vi "Set DataArray.vi"   [LabVIEW 2016, in "DataGrid.lvlib" / "DataGridView.lvclass"]
uses:
  <userlib>/LabVIEWdotNetDataGrid/source/DataGridView/DataGridView.lvclass
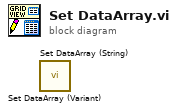
[diagram p0: block diagram]
diagram:
  n1 = call <userlib>:"Set DataArray (String).vi"() -> ()  [unwired: 10 in, 2 out]
  n2 = call <userlib>:"Set DataArray (Variant).vi"() -> ()  [unwired: 10 in, 2 out]
